vi "Get register for reading.vi"   [LabVIEW 2020, in "Toggle 8.lvclass"]
uses:
  Toggle 8.lvclass
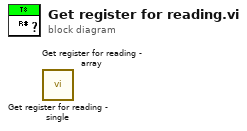
[diagram p0: block diagram]
diagram:
  n1 = call "Get register for reading - single.vi"() -> ()  [unwired: 11 in, 1 out]
  n2 = call "Get register for reading - array.vi"() -> ()  [unwired: 11 in, 1 out]
